vi "LCP Get No Of Pumps.vi"(8 "error in (no error)":errorcluster caption="Fehler (Eingang, kein Fehler)") -> (0 "error out":errorcluster caption="Fehler (Ausgang)", 3 "Pump Count":i32)   [LabVIEW 2023, in "labbCAN_Pump_API.lvlib"]
doc: "LCP_Func long LCP_CALL LCP_GetNoOfPumps();"
uses:
  labbCAN_Pump_API.lvlib
  labbCAN_Pump_API.dll
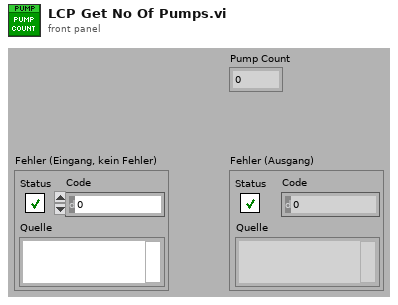
[diagram p1: front panel]
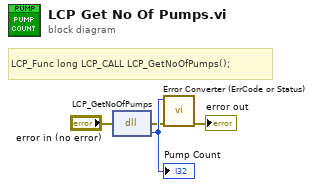
[diagram p0: block diagram]
diagram:
  # "LCP_Func long LCP_CALL LCP_GetNoOfPumps();"
  n1 = dll-call lib="C:/GIT/AutomatedSetupAcousticEnergyDensity/CETONI_SDK/labbCAN_Pump_API.*" fn="LCP_GetNoOfPumps"(error in="error in (no error)") -> (error out=w2:errorcluster, w4:i32)  [unwired: 2 in, 1 out]
  "Pump Count" <- w4
  n2 = call "Error Converter (ErrCode or Status).vi"("error in (no error)"=w2, "error code"=w4) -> ("error out"=→"error out":errorcluster)  [unwired: 9 in]
